vi "Test_Comm2.vi"() -> ()   [LabVIEW 2012]
uses:
  <vilib>/Platform/TimedLoop/XDataNode/XDataNode.xnode
  <vilib>/Platform/TimedLoop/XDataNode/nitl_modes.ctl
  <vilib>/Platform/TimedLoop/XDataNode/XDNodeRunTimeDep.lvlib
  <vilib>/Platform/TimedLoop/XDataNode/wakeup.ctl
  <vilib>/Platform/TimedLoop/XDataNode/timing_clust.ctl
panel:
  in  "Stop":bool
  out "timed out?":bool
  out "Error":errorcluster
  out "TimePressed":timestamp
  in  "On":bool
  out "error out":errorcluster
  out "RTTime":timestamp
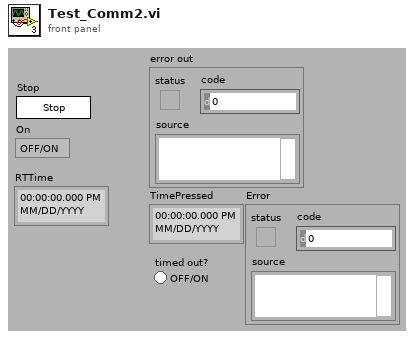
[diagram p1: front panel]
types:
  T1 = typedef "XDNodeRunTimeDep.lvlib/timing_clust.ctl" = cluster{"Expected End [f-1]":u64, "Actual End [f-1]":u64, "Finished Late? [f-1]":bool, "Expected End [i-1]":u64, "Actual End [i-1]":u64, "Finished Late? [i-1]":bool, "Expected Start [i]":u64, "Actual Start [i]":u64, "Expected Start [f]":u64, "Actual Start [f]":u64, "Source Name":string, "Structure Name":string, "Period":i64, "Deadline":i64, "Offset":i64, "Start":i64, "Priority":i32, "Timeout":i32, "Mode":T2, "Wakeup Reason":T3, "Error":errorcluster, "Source Type":string, "Secondary Source Type":string, "Global End Time":u64, "Global Start Time":u64, "Frame Duration":u64, "Iteration Duration":u64, "Assigned CPU":i32, "I/O Scan Engine Mode":u32}
  T2 = typedef "XDNodeRunTimeDep.lvlib/nitl_modes.ctl" = enum32{"No Change", "Process missed periods, maintain original phase", "Discard missed periods, maintain original phase", "Process missed periods, ignore original phase", "Discard missed periods, ignore original phase"}
  T3 = typedef "XDNodeRunTimeDep.lvlib/wakeup.ctl" = enum32{"Normal", "Aborted", "Asynchronous wakeup", "Timing source error", "Timed loop error", "Timeout"}
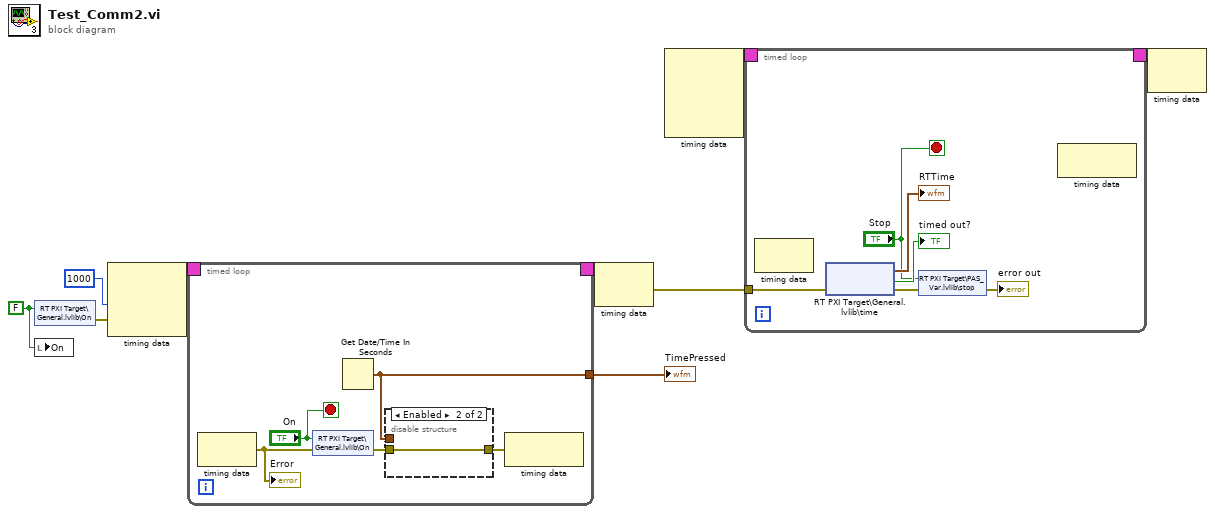
[diagram p0: block diagram]
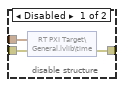
[diagram p2: hidden frame]
diagram:
  w3 = FALSE ("On")
  n1 = shared-variable "RT PXI Target\\General.lvlib\\On"(w3) -> (error out=w4:errorcluster)  [unwired: 1 in]
  n2 = local write "On"(w3) -> ()
  n3 = node-c288(i64 1000 ("Period"), w4) -> (w9:T1)  [unwired: 1 in]
  n4 = timed-loop {
    timing: w9 -> [_]
    timing-out: [_] -> w8
    tunnel: [w14] -> w5
    stop <- "On" stop-if-true
    n5 = node-c288() -> (w11:errorcluster)  [unwired: 1 in]
    "Error" <- w11
    n6 = shared-variable "RT PXI Target\\General.lvlib\\On"("On", error in=w11) -> (error out=w10:errorcluster)
    n7 = Get Date/Time In Seconds() -> (seconds since 1Jan1904=w14:timestamp)
    n8 = disable-structure shown="Enabled" {
      disable-tunnel: w14 -> [w17 _]
      disable-tunnel: [w16 w18] -> w13
      disable-tunnel: w10 -> [w15 w18]
      frame Disabled {
        n9 = shared-variable "RT PXI Target\\General.lvlib\\time"(w17, error in=w15) -> (error out=w16:errorcluster)
      }
      frame Enabled {
      }
    }
    n10 = node-c288(w13) -> ()  [unwired: 1 out]
  }
  "TimePressed" <- w5
  n11 = node-c288(w8) -> (w6:errorcluster)
  n12 = node-c288() -> (w2:T1)  [unwired: 4 in]
  n13 = timed-loop {
    tunnel: w6 -> [w28]
    timing: w2 -> [_]
    timing-out: [_] -> w1
    stop <- "Stop" stop-if-true
    n14 = node-c288() -> ()  [unwired: 1 in, 1 out]
    n15 = shared-variable "RT PXI Target\\General.lvlib\\time"(error in=w28) -> (→"RTTime":timestamp, error out=w25:errorcluster, →"timed out?":bool)  [unwired: 1 in]
    n16 = shared-variable "RT PXI Target\\PAS_Var.lvlib\\stop"("Stop", error in=w25) -> (error out=→"error out":errorcluster)
    n17 = node-c288() -> ()  [unwired: 1 in, 1 out]
  }
  n18 = node-c288(w1) -> ()  [unwired: 1 out]
